vi "ZPKtoSOS.vi"() -> ()   [LabVIEW 2011]
uses:
  <vilib>/addons/Digital Filter Design/_Objects.llb/DFD Filter Obj.ctl
  <vilib>/addons/Digital Filter Design/_Objects.llb/DFD Filter Coef.ctl
  <vilib>/addons/Digital Filter Design/_Objects.llb/DFD Filter Structure Type Selector.ctl
  <vilib>/addons/Digital Filter Design/_Objects.llb/dfd_Internal Quantization Settings.ctl
  <vilib>/addons/Digital Filter Design/_Objects.llb/dfd_Internal Quantization Srcs.ctl
  <vilib>/addons/Digital Filter Design/_Objects.llb/DFD Coef Norm Type.ctl
  <vilib>/addons/Digital Filter Design/_Objects.llb/DFD Output Iwl Obj.ctl
  <vilib>/addons/Digital Filter Design/_Objects.llb/DFD Quantization Settings.ctl
  <vilib>/addons/Digital Filter Design/_Objects.llb/DFD Quantization Sources.ctl
  <vilib>/addons/Digital Filter Design/_Objects.llb/DFD Round-off Mode.ctl
  <vilib>/addons/Digital Filter Design/FXPModel.llb/DFD FXP Quantize Coef (Advanced).vi
  <vilib>/addons/Digital Filter Design/NI_DigFilterLicensed.lvlib
panel:
  out "filter out":T1={"mSRate_Fs"=1.0, "mSRate_Version"="2.0", "mSRate_Comments"="", "mSRate_OrgCoef"={"type"=enum."Undefined", "gain"=1.0, "coef a (k)"=[], "coef b (v)"=[]}, "mSRate_CurCoef"={"type"=enum."Undefined", "gain"=1.0, "coef a (k)"=[], "coef b (v)"=[]}, "mSRate_Quantized?"=FALSE, "mSRate_QCoef"={"type"=enum."Undefined", "gain"=1.0, "coef a (k)"=[], "coef b (v)"=[]}, "mSRate_QSettings"=[], "mSRate_Order"=0, "mSRate_Scaling"={"mSRate_ScaleByPowerOf2?"=FALSE, "mSRate_ScaleType"=enum."No Norm"}} {"mSRate_QSettings"."source" items=["Coef a/k"=0, "Coef b/v"=7, "Input"=1, "Output"=2, "Multiplicand"=3, "Product"=4, "Sum"=5, "Delay"=6, "Gain"=8]}
  in  "iwl coeff a":i16=2
  in  "iwl coeff b":i16=2
  in  "wl":i16=22
  out "phase (deg)":cluster{"Y":dbl[], "Y":dbl[]}[](graph)
  out "gain (dB)":cluster{"Y":dbl[], "Y":dbl[]}[](graph)
  out "coeff b":dbl[](array[numeric])
  out "coeff a":dbl[](array[numeric])
  out "gain":dbl
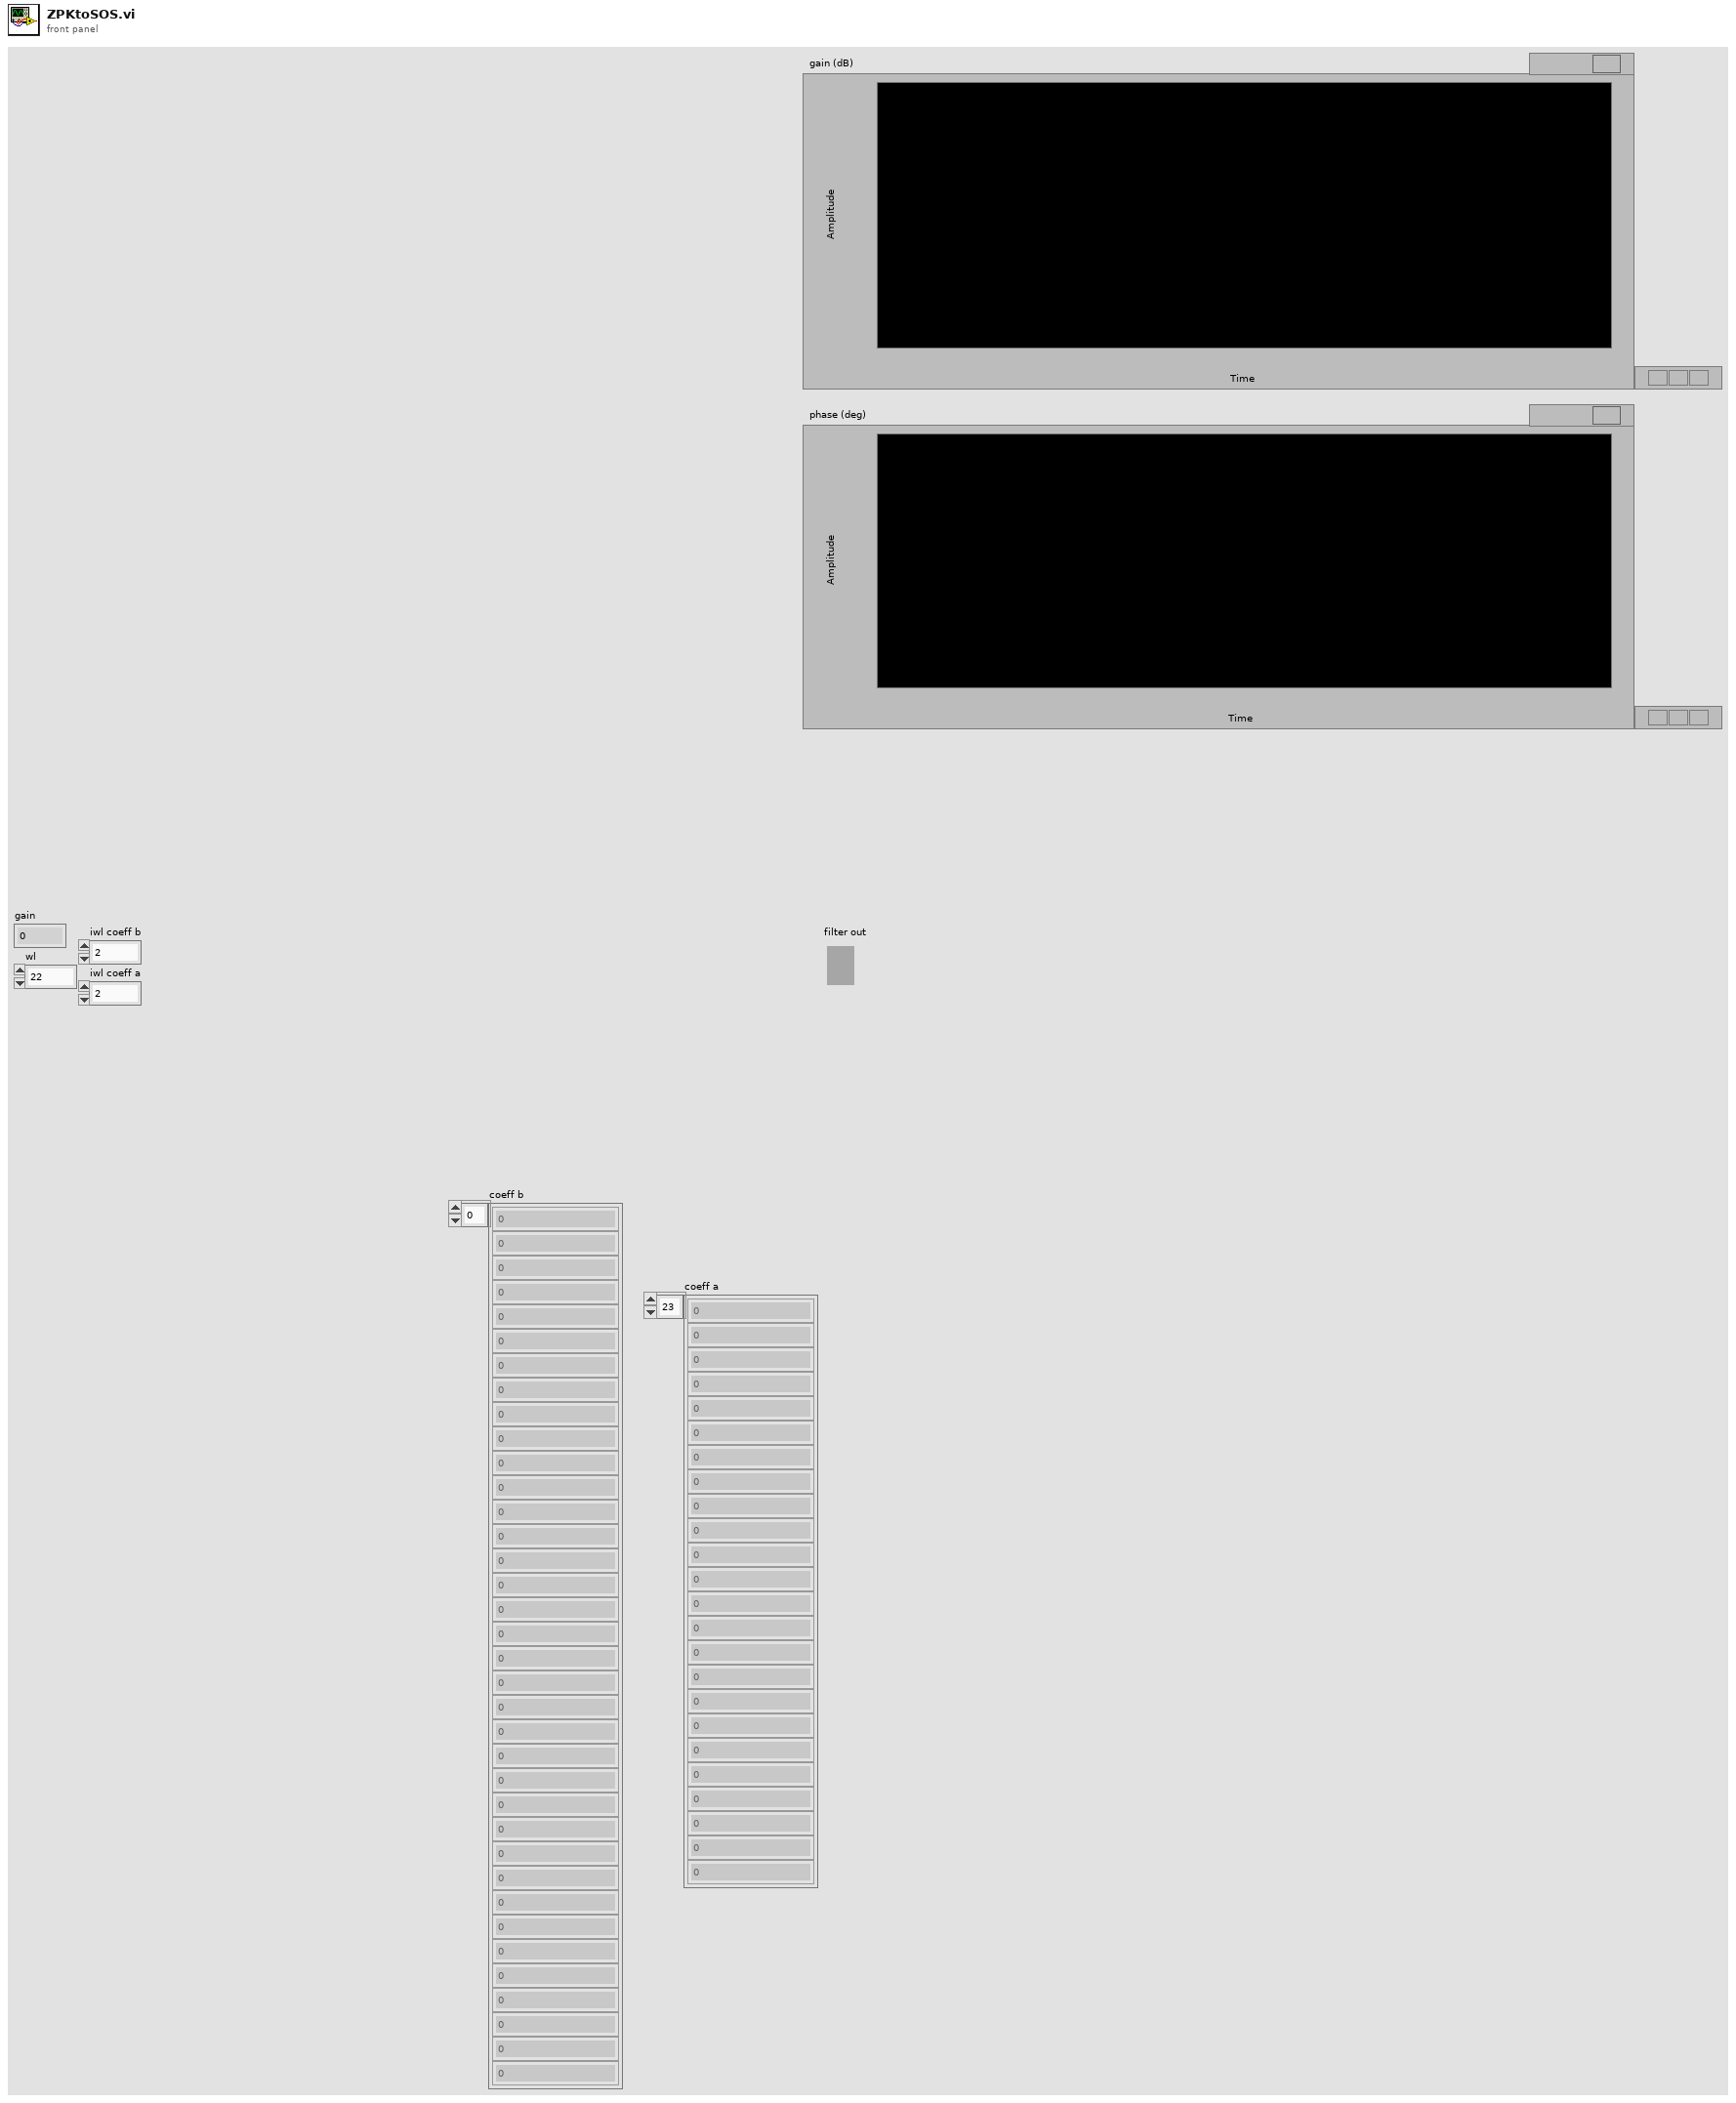
[diagram p1: front panel]
types:
  T1 = typedef "NI_DigFilterLicensed.lvlib/DFD Filter Obj.ctl" = cluster{"mSRate_Fs":dbl, "mSRate_Version":string, "mSRate_Comments":string, "mSRate_OrgCoef":T2, "mSRate_CurCoef":T2, "mSRate_Quantized?":bool, "mSRate_QCoef":T2, "mSRate_QSettings":T4[], "mSRate_Order":i32, "mSRate_Scaling":cluster{"mSRate_ScaleByPowerOf2?":bool, "mSRate_ScaleType":T6}}
  T2 = typedef "NI_DigFilterLicensed.lvlib/DFD Filter Coef.ctl" = cluster{"type":T3, "gain":dbl, "coef a (k)":dbl[], "coef b (v)":dbl[]}
  T3 = typedef "NI_DigFilterLicensed.lvlib/DFD Filter Structure Type Selector.ctl" = enum16{"Undefined", "FIR Direct Form", "FIR Direct Form Transposed", "FIR Symmetric", "FIR Antisymmetric", "IIR Direct Form I", "IIR Direct Form I Transposed", "IIR Direct Form II", "IIR Direct Form II Transposed", "IIR Cascaded Second Order Sections Form I", "IIR Cascaded Second Order Sections Form I Transposed", "IIR Cascaded Second Order Sections Form II", "IIR Cascaded Second Order Sections Form II Transposed", "Lattice Allpass (basic sections)", "Lattice Allpass (one multiplier sections)", "Lattice Allpass (normalized sections)", "Lattice AR (basic sections)", "Lattice AR (one multiplier sections)", "Lattice AR (normalized sections)", "Lattice MA (minimum phase)", "Lattice MA (maximum phase)", "Lattice ARMA (basic sections)", "Lattice ARMA (one multiplier sections)", "Lattice ARMA (normalized sections)"}
  T4 = typedef "NI_DigFilterLicensed.lvlib/dfd_Internal Quantization Settings.ctl" = cluster{"source":T5, "wl":i16, "iwl":i16, "overflow mode":enum16{"Saturation", "Wrap"}, "rounding mode":enum16{"Nearest", "Truncation"}, "signed?":bool}
  T5 = typedef "NI_DigFilterLicensed.lvlib/dfd_Internal Quantization Srcs.ctl" = u16
  T6 = typedef "NI_DigFilterLicensed.lvlib/DFD Coef Norm Type.ctl" = enum16{"No Norm", "Time Domain 1-Norm", "Time Domain 2-Norm", "Time Domain Inf-Norm"}
  T7 = typedef "NI_DigFilterLicensed.lvlib/DFD Round-off Mode.ctl" = enum16{"Nearest", "Truncation"}
  T8 = typedef "NI_DigFilterLicensed.lvlib/DFD Quantization Settings.ctl" = cluster{"source":T9, "wl":i16, "iwl":i16, "overflow mode":enum16{"Saturation", "Wrap"}, "rounding mode":enum16{"Nearest", "Truncation"}, "signed?":bool}
  T9 = typedef "NI_DigFilterLicensed.lvlib/DFD Quantization Sources.ctl" = u16
  T10 = typedef "NI_DigFilterLicensed.lvlib/DFD Output Iwl Obj.ctl" = cluster{"output option":enum16{"Auto", "Same As Input", "User Defined"}, "integer word length":i16}
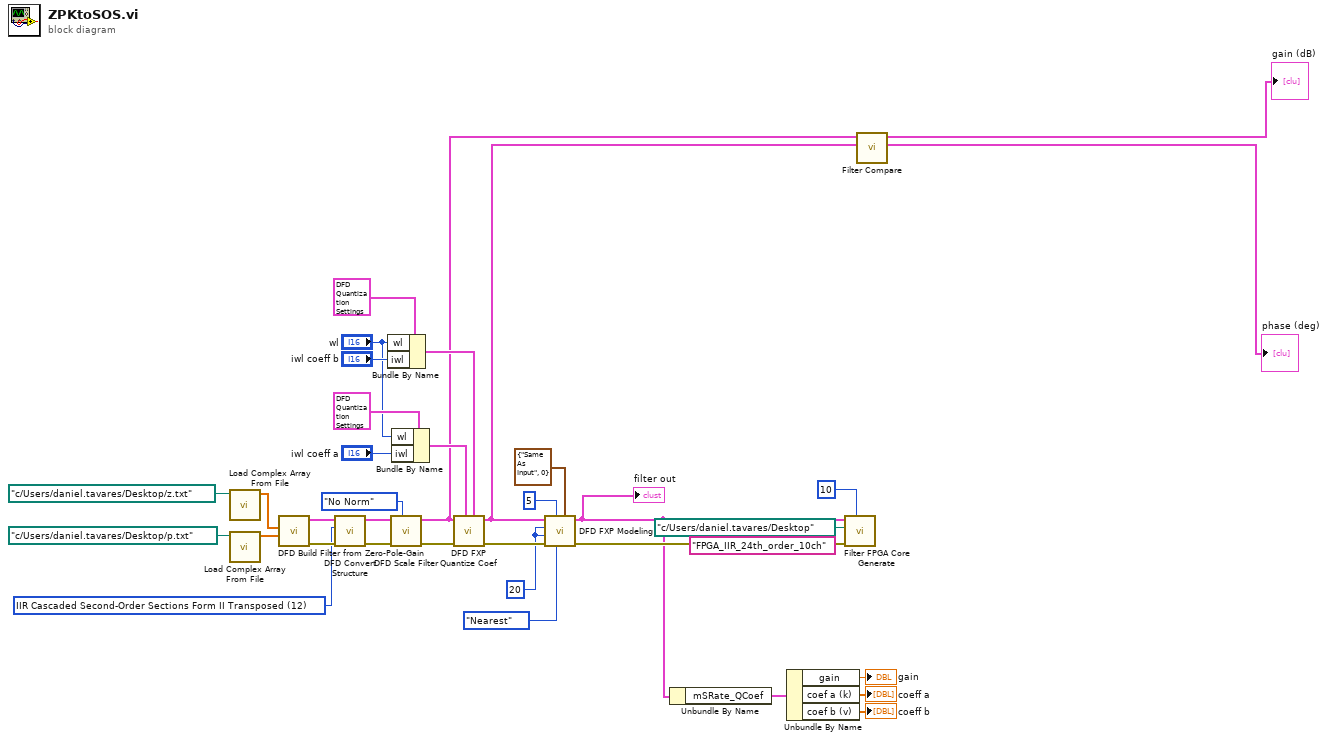
[diagram p0: block diagram]
diagram:
  w27 = i16 20 ("input word length")
  w34 = u16 12 items=["FIR Direct Form"=1, "FIR Direct Form Transposed"=2, "FIR Symmetric"=3, "FIR Antisymmetric"=4, "IIR Direct Form I"=5, "IIR Direct Form I Transposed"=6, "IIR Direct Form II"=7, "IIR Direct Form II Transposed"=8, "IIR Cascaded Second-Order Sections Form I"=9, "IIR Cascaded Second-Order Sections Form I Transposed"=10, "IIR Cascaded Second-Order Sections Form II"=11, "IIR Cascaded Second-Order Sections Form II Transposed"=12, "Lattice Allpass (basic sections)"=13, "Lattice Allpass (one multiplier sections)"=14, "Lattice Allpass (normalized sections)"=15, "Lattice AR (basic sections)"=16, "Lattice AR (one multiplier sections)"=17, "Lattice AR (normalized sections)"=18, "Lattice MA (minimum phase)"=19, "Lattice MA (maximum phase)"=20, "Lattice ARMA (basic sections)"=21, "Lattice ARMA (one multiplier sections)"=22, "Lattice ARMA (normalized sections)"=23] ("target structure")
  n1 = call "Load Complex Array From File.vi"("file path (dialog if empty)"=path "c:/Users/daniel.tavares/Desktop/z.txt") -> ("Array"=w6:cdb[])  [unwired: 10 in]
  n2 = call "Load Complex Array From File.vi"("file path (dialog if empty)"=path "c:/Users/daniel.tavares/Desktop/p.txt") -> ("Array"=w8:cdb[])  [unwired: 10 in]
  n3 = call <vilib>:"DFD Build Filter from Zero-Pole-Gain.vi"("poles"=w8, "zeroes"=w6) -> ("error out"=w35:errorcluster, "filter out"=w29:T1)  [unwired: 8 in]
  n4 = call <vilib>:"DFD Convert Structure.vi"("error in (no error)"=w35, "target structure"=w34, "filter in"=w29) -> ("error out"=w16:errorcluster, "filter out"=w17:T1)  [unwired: 7 in]
  n5 = Bundle By Name(cluster=T8 {"source"=7, "wl"=20, "iwl"=1, "overflow mode"=enum."Saturation", "rounding mode"=enum."Nearest", "signed?"=TRUE} ("coefficients b/v quantizer"), "wl"="wl", "iwl"="iwl coeff b") -> (w20:T8)
  n6 = call <vilib>:"DFD Scale Filter.vi"("scale type"=DFD_Coef_Norm_Type."No Norm", "error in (no error)"=w16, "filter in"=w17) -> ("error out"=w15:errorcluster, "filter out"=w13:T1)  [unwired: 7 in]
  n7 = Bundle By Name(cluster=T8 {"source"=0, "wl"=20, "iwl"=1, "overflow mode"=enum."Saturation", "rounding mode"=enum."Nearest", "signed?"=TRUE} ("coefficients a/k quantizer"), "wl"="wl", "iwl"="iwl coeff a") -> (w19:T8)
  n8 = call-poly <vilib>:"DFD FXP Quantize Coef.vi"("coefficients b/v quantizer"=w20, "coefficients a/k quantizer"=w19, "error in (no error)"=w15, "filter in"=w13) -> ("error out"=w33:errorcluster, "filter out"=w12:T1)  [unwired: 6 in]
  n9 = call <vilib>:"DFD FXP Modeling.vi"("output integer word length"=T10 {"output option"=enum."Same As Input", "integer word length"=0}, "output rounding mode"=DFD_Round-off_Mode."Nearest", "input integer word length"=i16 5, "error in (no error)"=w33, "output word length"=w27, "input word length"=w27, "filter in"=w12) -> ("error out"=w36:errorcluster, "filter out"=w25:T1)  [unwired: 3 in]
  "filter out" <- w25
  n10 = Unbundle By Name(w25) -> ("mSRate_QCoef"=w32:T2)
  n11 = Unbundle By Name(w32) -> ("gain"=→"gain":dbl, "coef a (k)"=→"coeff a":dbl[], "coef b (v)"=→"coeff b":dbl[])
  n12 = call "Filter FPGA Core Generate.vi"("# channels"=10, "error in (no error)"=w36, "filter name"="FPGA_IIR_24th_order_10ch", "destination folder"=path "c:/Users/daniel.tavares/Desktop", "filter"=w25) -> ()  [unwired: 6 in, 1 out]
  n13 = call "Filter Compare.vi"("quantized filter"=w12, "filter"=w13) -> ("phase (deg)"=→"phase (deg)":cluster{"Y":dbl[], "Y":dbl[]}[], "gain (dB)"=→"gain (dB)":cluster{"Y":dbl[], "Y":dbl[]}[])  [unwired: 8 in]
